vi "Temp scan setup.vi"(7 "VISA resource name":refnum<visa-resource-name>="GPIB0::16::INSTR", 8 "error in (no error)":errorcluster caption="错误输入（无错误）", 9 "Sample Count (100)":i32=100, 10 "Channel List (101:110)":string, 11 "2700 输入":refnum<class "2700.lvclass">) -> (0 "error out":errorcluster caption="错误输出", 3 "2700 输出":refnum<class "2700.lvclass">)   [LabVIEW 2021, in "2700.lvclass"]
uses:
  2700.lvclass
  2700.lvclass/2700.ctl
  <instrlib>/Keithley 27XX/Public/Configure/Measurement Specific/Configure Thermocouple.vi
  <instrlib>/Keithley 27XX/Keithley 27XX.lvlib
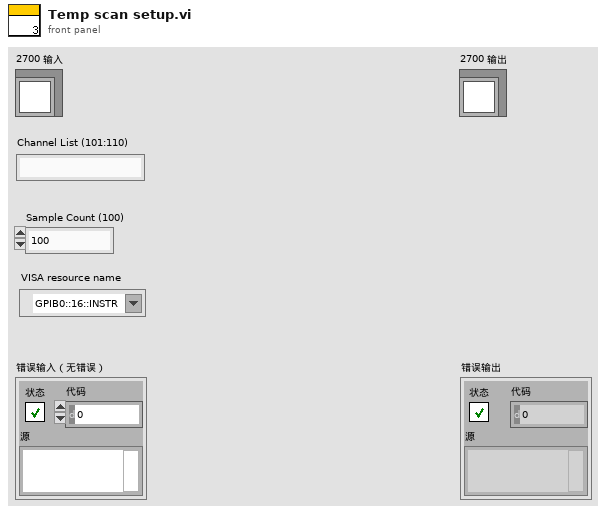
[diagram p1: front panel]
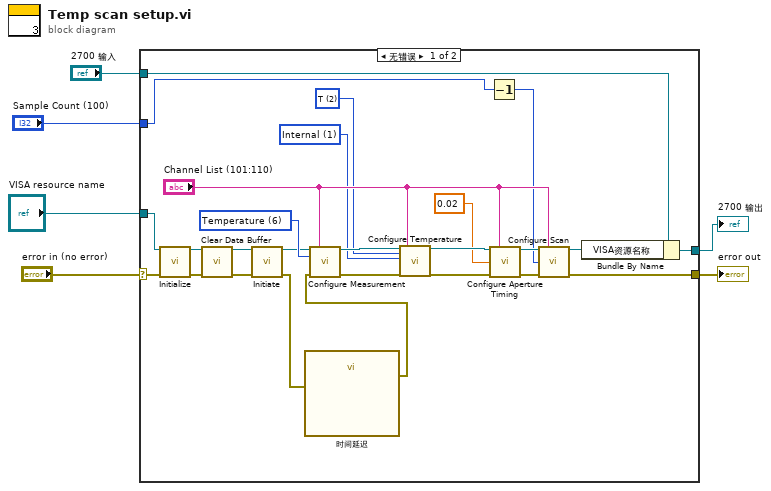
[diagram p0: block diagram]
diagram:
  n1 = case shown="无错误" "error in (no error)" {
    selector: "error in (no error)" -> [w21 w33]
    tunnel: "2700 输入" -> [w19 w34]
    tunnel: "Sample Count (100)" -> [w16 _]
    tunnel: [w18 w34] -> w3
    tunnel: [w9 w33] -> w2
    tunnel: "VISA resource name" -> [w20 _]
    frame No Error {
      w22 = u16 1 items=["Simulated", "Internal", "External"] ("Reference Junction Type (0: Simulated)")
      w23 = u16 2 items=["J", "K", "T", "E", "R", "S", "B", "N"] ("Thermocouple Type (1: K)")
      w24 = u16 6 items=["DC Voltage", "AC Voltage", "DC Current", "AC Current", "Resistance", "Four-Wire Resistance", "Temperature", "Frequency", "Period", "Continuity"] ("Function (0: DC Voltage)")
      n2 = call <instrlib>:"Initialize.vi"("VISA resource name"=w20, "error in (no error)"=w21) -> ("VISA resource name out"=w14:refnum<visa-resource-name>, "error out"=w15:errorcluster)  [unwired: 12 in]
      n3 = call <instrlib>:"Clear Data Buffer.vi"("VISA resource name"=w14, "error in (no error)"=w15) -> ("VISA resource name out"=w12:refnum<visa-resource-name>, "error out"=w11:errorcluster)  [unwired: 12 in]
      n4 = call <instrlib>:"Initiate.vi"("VISA resource name"=w12, "error in (no error)"=w11) -> ("VISA resource name out"=w13:refnum<visa-resource-name>, "error out"=w8:errorcluster)  [unwired: 12 in]
      n5 = call "时间延迟"("error in (no error)"=w8) -> ("error out"=w7:errorcluster)  [unwired: 10 in]
      n6 = call <instrlib>:"Configure Measurement.vi"("VISA resource name"=w13, "Scan List (Empty)"="Channel List (101:110)", "Function (0: DC Voltage)"=w24, "error in (no error)"=w7) -> ("VISA resource name out"=w26:refnum<visa-resource-name>, "error out"=w27:errorcluster)  [unwired: 10 in]
      n7 = call-poly <instrlib>:"Configure Temperature.vi"("VISA resource name"=w26, "Thermocouple Type (1: K)"=w23, "Reference Junction Type (0: Simulated)"=w22, "error in (no error)"=w27, "Scan List (Empty)"="Channel List (101:110)") -> ("VISA resource name out"=w29:refnum<visa-resource-name>, "error out"=w28:errorcluster)  [unwired: 13 in]
      n8 = Decrement(x=w16) -> (x-1=w17:i32)
      n9 = call <instrlib>:"Configure Aperture Timing.vi"("VISA resource name"=w29, "Scan List (Empty)"="Channel List (101:110)", "Timing Value (0.020)"=0.02, "error in (no error)"=w28) -> ("VISA resource name out"=w31:refnum<visa-resource-name>, "error out"=w32:errorcluster)  [unwired: 10 in]
      n10 = call <instrlib>:"Configure Scan.vi"("VISA resource name"=w31, "Channel List (101:110)"="Channel List (101:110)", "Sample Count (100)"=w17, "error in (no error)"=w32) -> ("VISA resource name out"=w10:refnum<visa-resource-name>, "error out"=w9:errorcluster)  [unwired: 10 in]
      n11 = Bundle By Name(cluster=w19, "VISA资源名称"=w10) -> (w18:refnum<class "2700.lvclass">)
    }
    frame Error {
    }
  }
  "error out" <- w2
  "2700 输出" <- w3
